vi "Configure.vi"(8 "error in (no error)":errorcluster, 9 "Value in":u8, 10 "Use Counter?":bool, 11 "Loopback in":refnum<class "Loopback.lvclass">) -> (0 "error out":errorcluster, 3 "Loopback out":refnum<class "Loopback.lvclass">)   [LabVIEW 2016, in "Loopback.lvclass"]
uses:
  Loopback.lvclass
  Loopback.lvclass/Loopback.ctl
  <vilib>/Utility/error.llb/Error Cluster From Error Code.vi
  <vilib>/rvi/errors/niLvFpgaAdjustHostInterfaceError.vi
  <vilib>/rvi/interface/nirviReadWriteControl/nirviReadWriteControl.xnode
  NiFpgaLv.dll
  <vilib>/rvi/interface/Simulation/niFpgaSimulationCallBeginRW.vi
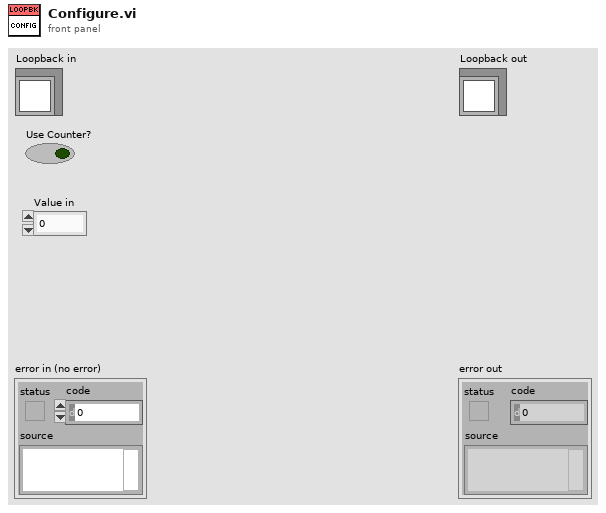
[diagram p1: front panel]
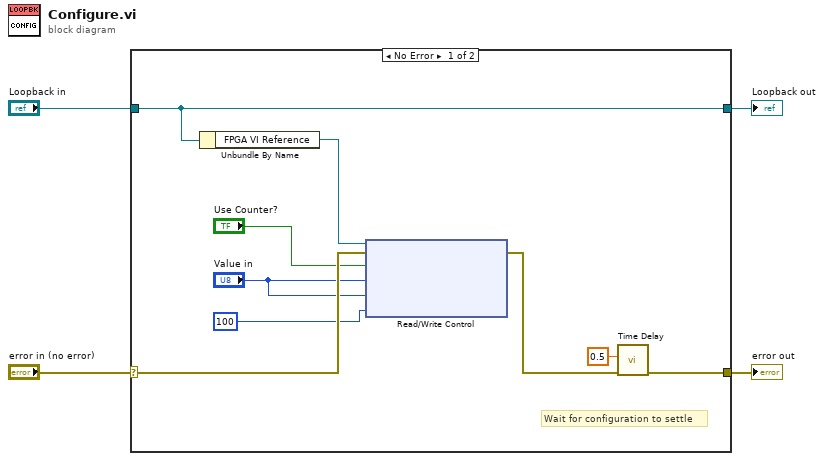
[diagram p0: block diagram]
diagram:
  n1 = case shown="No Error" "error in (no error)" {
    selector: "error in (no error)" -> [w9 w15]
    tunnel: [w8 w15] -> w3
    tunnel: [w11 w14] -> w1
    tunnel: "Loopback in" -> [w11 w14]
    frame No Error {
      # "Wait for configuration to settle"
      n2 = Unbundle By Name(w11) -> ("FPGA VI Reference"=w10:refnum<k20>)
      n3 = xnode "Read/Write Control"("FPGA VI Reference In"=w10, "error in"=w9, "Use Counter?"="Use Counter?", "Connector0/DIOPORT3"="Value in", "Connector0/DIOPORT0"="Value in", "Wait (mSec)"=u32 100) -> ("error out"=w13:errorcluster)  [unwired: 1 out]
      n4 = call "Time Delay"("error in (no error)"=w13, "Delay Time (s)"=0.5) -> ("error out"=w8:errorcluster)  [unwired: 9 in]
    }
    frame Error {
    }
  }
  "error out" <- w3
  "Loopback out" <- w1
